vi "Reset Mode FGV.vi"(8 "Error In":errorcluster) -> (0 "Error Out":errorcluster)   [LabVIEW 2014]
uses:
  Web Services/DronePi Global Variables.vi
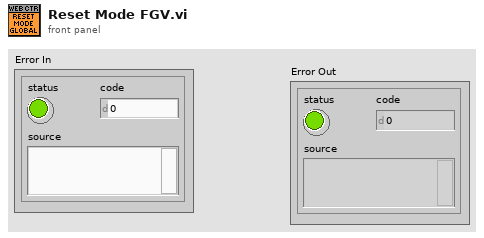
[diagram p1: front panel]
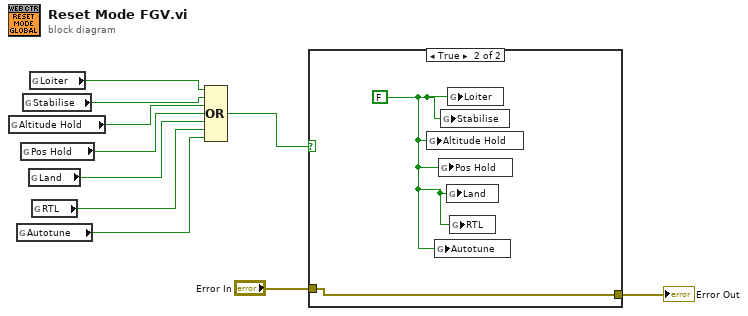
[diagram p0: block diagram]
diagram:
  n1 = global read "DronePi Global Variables.vi" "Altitude Hold"() -> (w8:bool)
  n2 = global read "DronePi Global Variables.vi" "Autotune"() -> (w4:bool)
  n3 = global read "DronePi Global Variables.vi" "Pos Hold"() -> (w7:bool)
  n4 = global read "DronePi Global Variables.vi" "Stabilise"() -> (w9:bool)
  n5 = global read "DronePi Global Variables.vi" "Land"() -> (w6:bool)
  n6 = global read "DronePi Global Variables.vi" "Loiter"() -> (w10:bool)
  n7 = global read "DronePi Global Variables.vi" "RTL"() -> (w5:bool)
  n8 = Compound Arithmetic op=OR(w10, w9, w8, w7, w6, w5, w4) -> (w3:bool)
  n9 = case shown="True" w3 {
    tunnel: "Error In" -> [w11 w12]
    tunnel: [w11 w12] -> w1
    frame False {
    }
    frame True {
      w13 = FALSE ("Loiter")
      n10 = global write "DronePi Global Variables.vi" "Altitude Hold"(w13) -> ()
      n11 = global write "DronePi Global Variables.vi" "Autotune"(w13) -> ()
      n12 = global write "DronePi Global Variables.vi" "Pos Hold"(w13) -> ()
      n13 = global write "DronePi Global Variables.vi" "Stabilise"(w13) -> ()
      n14 = global write "DronePi Global Variables.vi" "Land"(w13) -> ()
      n15 = global write "DronePi Global Variables.vi" "Loiter"(w13) -> ()
      n16 = global write "DronePi Global Variables.vi" "RTL"(w13) -> ()
    }
  }
  "Error Out" <- w1
